vi "base sensor interrupt.vi"(11 "IRQ Number":u8) -> ()   [LabVIEW 2015]
uses:
  <vilib>/myRIO/Common/Instrument Driver Framework/myRIO v1.0/myRIO v1.0 Close.vi
  <vilib>/myRIO/Common/Instrument Driver Framework/Utilities/vis/FPGA Ref Manager.vi
  <vilib>/myRIO/Common/Instrument Driver Framework/myRIO v1.0/IRQ/vis/myRIO v1.0 Reserve IRQ.vi
  ARM angles.vi
  <vilib>/myRIO/Instrument Drivers/IRQ/IO IRQ/IO IRQ.lvlib
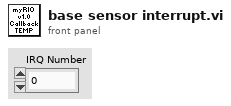
[diagram p1: front panel]
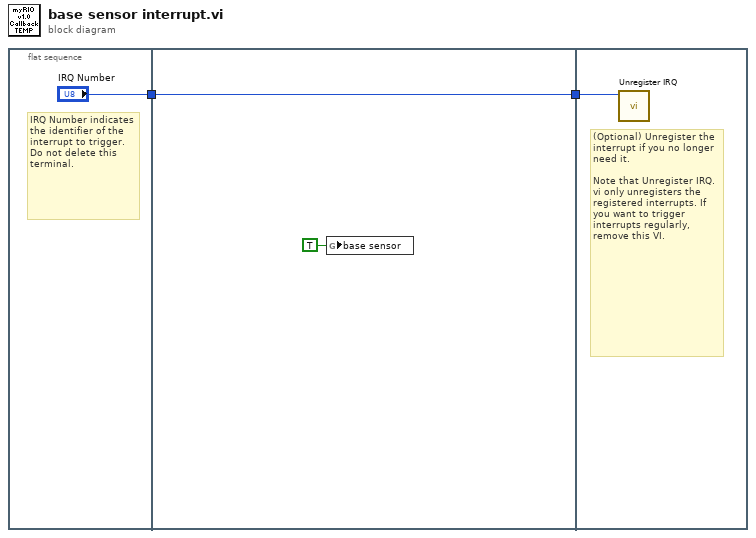
[diagram p0: block diagram]
diagram:
  n1 = flat-sequence {
    tunnel: ["IRQ Number"] -> w2
    tunnel: [w5] -> w1
    tunnel: w2 -> [w5]
    tunnel: w1 -> [w6]
    frame #0 {
      # "IRQ Number indicates the identifier of the interrupt to trigger. Do not delete this terminal."
    }
    frame #1 {
      n2 = global write "ARM angles.vi" "base sensor"(TRUE ("base sensor")) -> ()
    }
    frame #2 {
      # "(Optional) Unregister the interrupt if you no longer need it.\n\nNote that Unregister IRQ.vi only unregisters the registered interrupts. If you want to trigger interrupts regularly, remove this VI."
      n3 = call <vilib>:"Unregister IRQ.vi"("IRQ Number"=w6) -> ()  [unwired: 10 in, 1 out]
    }
  }
